vi "Maui 2.0. Set Subpanels.SMO Array.vi"(6 "Append (F)":bool, 8 "error in (no error)":errorcluster, 10 "Subpanels in":refnum<class "SMO.lvclass">[](array[class]), 11 "Maui 2.0 in":refnum<class "Maui 2.0.lvclass">) -> (0 "error out":errorcluster, 2 "Subpanels Out":refnum<class "SMO.lvclass">[](array[class]), 3 "Maui 2.0 out":refnum<class "Maui 2.0.lvclass">)   [LabVIEW 2020, in "Maui 2.0.lvclass"]
uses:
  Maui 2.0.lvclass
  <vilib>/JKI/JKI SMO/SMO/SMO.lvclass
  Typedefs/PrivateEvents--Maui 2.0.Set Subpanels.ctl
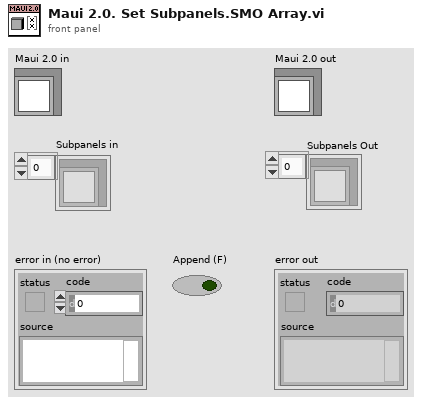
[diagram p1: front panel]
types:
  T1 = typedef "Maui 2.0.lvclass/PrivateEvents--Maui 2.0.Set Subpanels.ctl" = cluster{"Subpanels":refnum<class "SMO.lvclass">[], "Append":bool}
  T2 = typedef "SMO.lvclass/SMOState --Enum.ctl" = enum16{"unknown", "Created", "Started", "Stopped"}
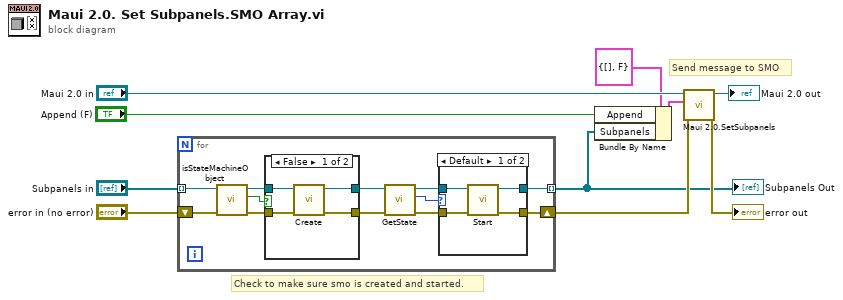
[diagram p0: block diagram]
diagram:
  # "Send message to SMO"
  # "Check to make sure smo is created and started."
  n1 = for {
    tunnel: "Subpanels in" -> [w22] mode=indexing
    shift-right: [w12] -> w6
    shift-left: "error in (no error)" -> [w13]
    tunnel: [w11] -> w2 mode=indexing
    n2 = call <vilib>:"isStateMachineObject.vi"("error in (no error)"=w13, "SMO"=w22) -> ("error out"=w20:errorcluster, "is SMO?"=w15:bool, "SMO out"=w21:refnum<class "SMO.lvclass">)  [unwired: 7 in]
    n3 = case shown="False" w15 {
      tunnel: w21 -> [w32 w34]
      tunnel: w20 -> [w31 w33]
      tunnel: [w30 w34] -> w19
      tunnel: [w29 w33] -> w18
      frame False {
        n4 = call <vilib>:"Create.vi"("error in (no error)"=w31, "SMO"=w32) -> ("error out"=w29:errorcluster, "SMO out"=w30:refnum<class "SMO.lvclass">)  [unwired: 7 in, 1 out]
      }
      frame True {
      }
    }
    n5 = call <vilib>:"GetState.vi"("error in (no error)"=w18, "SMO"=w19) -> ("error out"=w16:errorcluster, "SMO State"=w14:T2, "SMO out"=w17:refnum<class "SMO.lvclass">)  [unwired: 7 in]
    n6 = case shown="Default" w14 {
      tunnel: w17 -> [w26 w28]
      tunnel: w16 -> [w25 w27]
      tunnel: [w24 w27] -> w12
      tunnel: [w23 w28] -> w11
      frame Default {
        n7 = call <vilib>:"Start.vi"("error in (no error)"=w25, "SMO"=w26) -> ("error out"=w24:errorcluster, "SMO out"=w23:refnum<class "SMO.lvclass">)  [unwired: 8 in]
      }
      frame "Started" {
      }
    }
  }
  "Subpanels Out" <- w2
  n8 = Bundle By Name(cluster=T1 {"Subpanels"=[], "Append"=FALSE} ("Set Subpanels"), "Append"="Append (F)", "Subpanels"=w2) -> (w3:T1)
  n9 = call "Maui 2.0.SetSubpanels.vi"("error in (no error)"=w6, "Set Subpanels"=w3, "Maui 2.0"="Maui 2.0 in") -> ("error out"=→"error out":errorcluster, "Maui 2.0 out"=→"Maui 2.0 out":refnum<class "Maui 2.0.lvclass">)  [unwired: 7 in]
